vi "Read_Data_MsgQ.vi"(6 "timeout in ms (10)":i32=10, 8 "error in (no error)":errorcluster) -> (0 "error out":errorcluster, 1 "timed out?":bool, 2 "Data out":string[](array[string]), 3 "ResponseAddr":string, 5 "Command out":T1)   [LabVIEW 2019, in "MsgQ.lvlib"]
uses:
  MsgQ.lvlib
  TypeDefs/MsgQ_Commands.ctl
  TypeDefs/CommandsQ.ctl
  Service/Service.lvlib
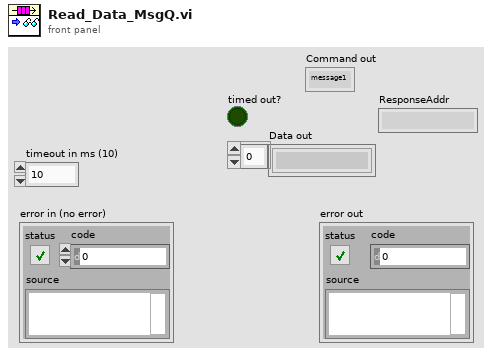
[diagram p1: front panel]
types:
  T1 = typedef "MsgQ.lvlib/MsgQ_Commands.ctl" = enum16{"message1", "message2", "message3", "generic", "transparent", "exception", "stop"}
  T2 = typedef "Service.lvlib/CommandsQ.ctl" = cluster{"cmd":T1, "data":variant, "notif":string}
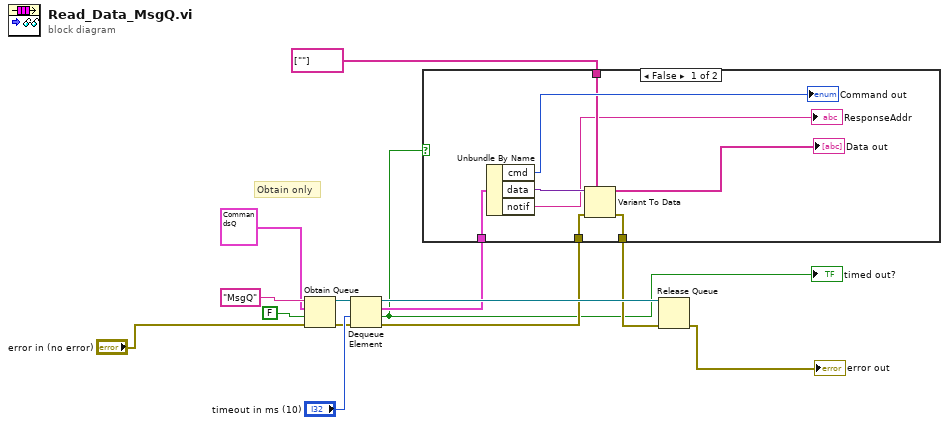
[diagram p0: block diagram]
diagram:
  # "Obtain only"
  n1 = Obtain Queue(name (unnamed)="MsgQ", element data type=T2 {"cmd"=enum."message1", "data"=variant, "notif"="notif1"}, create if not found? (T)=FALSE, error in (no error)="error in (no error)") -> (queue out=w10:refnum<queue>, error out=w6:errorcluster)  [unwired: 1 in, 1 out]
  n2 = Dequeue Element(queue=w10, timeout in ms (-1)="timeout in ms (10)", error in (no error)=w6) -> (queue out=w9:refnum<queue>, element=w5:T2, timed out?=w1:bool, error out=w3:errorcluster)
  "timed out?" <- w1
  n3 = case shown="False" w1 {
    tunnel: w5 -> [w22 _]
    tunnel: string[] [""] ("Data in") -> [w19 _]
    tunnel: w3 -> [w18 w23]
    tunnel: [w17 w23] -> w2
    frame False {
      n4 = Unbundle By Name(w22) -> ("cmd"=→"Command out":T1, "data"=w21:variant, "notif"=→"ResponseAddr":string)
      n5 = Variant To Data(error in=w18, type=w19, Variant=w21) -> (data=→"Data out":string[], error out=w17:errorcluster)
    }
    frame True {
    }
  }
  n6 = Release Queue(queue=w9, error in (no error)=w2) -> (error out=→"error out":errorcluster)  [unwired: 1 in, 2 out]
